vi "createController.vi"(8 "error in (no error)":errorcluster, 11 "Boot in":refnum<class "Boot.lvclass">) -> (0 "error out":errorcluster, 2 "Controller":refnum<class "Controller.lvclass">, 3 "Boot out":refnum<class "Boot.lvclass">)   [LabVIEW 2016, in "Boot.lvclass"]
uses:
  Boot.lvclass
  Controller/Controller.lvclass
  Boot.lvclass/Boot.ctl
  Controller/Controller.lvclass/Controller.ctl
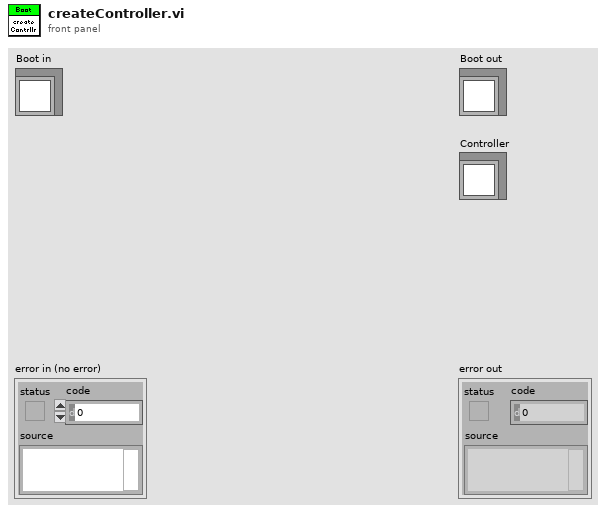
[diagram p1: front panel]
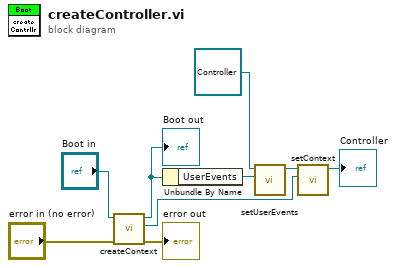
[diagram p0: block diagram]
diagram:
  n1 = call "createContext.vi"("error in (no error)"="error in (no error)", "Boot in"="Boot in") -> ("error out"=→"error out":errorcluster, "Context"=w3:refnum<class "Context.lvclass">, "Boot out"=w4:refnum<class "Boot.lvclass">)  [unwired: 7 in]
  "Boot out" <- w4
  n2 = Unbundle By Name(w4) -> ("UserEvents"=w7:refnum<class "UserEvents.lvclass">)
  n3 = call "setUserEvents.vi"("UserEvents"=w7, "Controller in"=refnum<class "Controller.lvclass"> refnum ("Controller.lvclass")) -> ("Controller out"=w8:refnum<class "Controller.lvclass">)  [unwired: 9 in]
  n4 = call "setContext.vi"("Context"=w3, "Controller in"=w8) -> ("Controller out"=→"Controller":refnum<class "Controller.lvclass">)  [unwired: 9 in]
